vi "Get Message Transport Singleton.vi"(8 "error in (no error)":errorcluster, 11 "Message Transport Singleton in":refnum<class "Message Transport Singleton.lvclass">=refnum) -> (0 "error out":errorcluster, 3 "Singleton Ref":refnum<data-value>)   [LabVIEW 2016, in "Stream Mediator.lvlib" / "Message Transport Singleton.lvclass"]
doc: "--\nCopyright © 2017 Composed SystemsI All rights reserved.\n\nAuthor: Jon McBee <jon.mcbee@composed.io>\n\nThis library is provided \"AS IS\" ,WITHOUT WARRANTIES OR\nCONDITIONS OF ANY KIND, either express or implied.\n\nComposed Systems -- composed.io\n\nStream 0.0.1.1\nJon McBee - Composed Systems\nCopyright (c) 2017, Composed Systems"
uses:
  <userlib>/Composed Systems/Stream/Mediator/Classes/Message Transport Singleton/Message Transport Singleton.lvclass
  <userlib>/Composed Systems/Stream/Mediator/Classes/Message Transport Singleton/Message Transport Singleton.lvclass/Message Transport Singleton.ctl
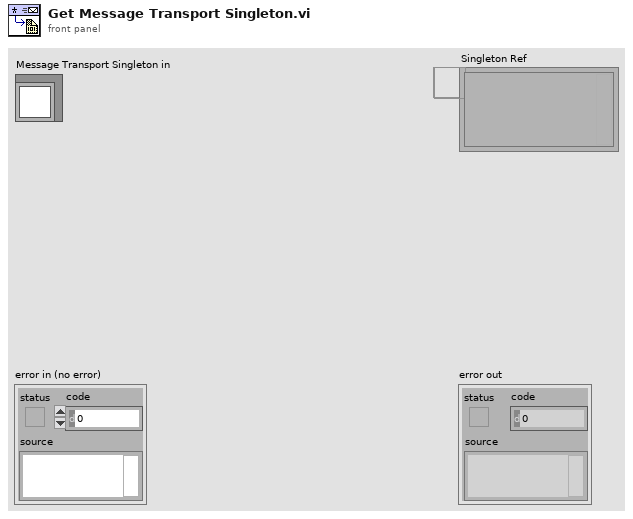
[diagram p1: front panel]
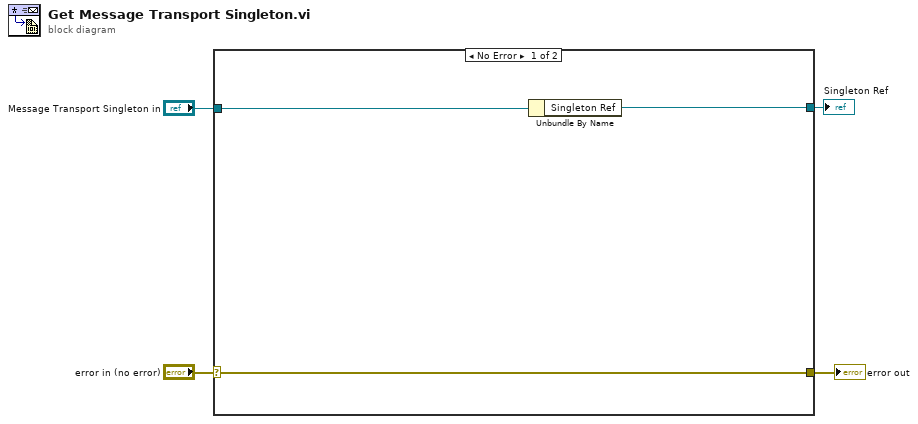
[diagram p0: block diagram]
diagram:
  n1 = case shown="No Error" "error in (no error)" {
    selector: "error in (no error)" -> [w7 w8]
    tunnel: [w7 w8] -> w3
    tunnel: "Message Transport Singleton in" -> [w6 _]
    tunnel: [w5 _] -> w1
    frame No Error {
      n2 = Unbundle By Name(w6) -> ("Singleton Ref"=w5:refnum<data-value>)
    }
    frame Error {
    }
  }
  "error out" <- w3
  "Singleton Ref" <- w1
